vi "Create Minor Frame Name from Rate.vi"(11 "rate":string) -> (3 "minor frame name out":string)   [LabVIEW 2020, in "Configuration_Helper.lvlib"]
uses:
  Configuration_Helper.lvlib
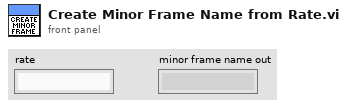
[diagram p1: front panel]
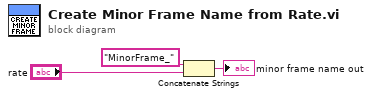
[diagram p0: block diagram]
diagram:
  n1 = Concatenate Strings("MinorFrame_" ("string"), "rate") -> (→"minor frame name out":string)
